vi "DHE_CheckShutDown.vi"() -> ()   [LabVIEW 2016]
panel:
  in  "cmds":string[](array[string])
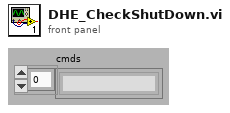
[diagram p1: front panel]
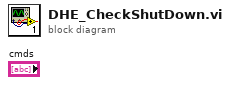
[diagram p0: block diagram]
diagram:
